vi "ProcessRun.vi"(5 "EndTime":timestamp, 7 "StartTime":timestamp, 8 "error in":errorcluster, 11 "ProcessRun":refnum<class "ProcessRun.lvclass">) -> (0 "error out":errorcluster, 3 "Passed":bool)   [LabVIEW 2020]
uses:
  ProligentResultProcessor/ProcessRun/ProcessRun.lvclass
  ProligentResultProcessor/ProcessRun/SetProcessRunId.vi
  ProligentResultProcessor/ProcessRun/SetProcessFullName.vi
  ProligentResultProcessor/ProcessRun/SetProcessVersion.vi
  ProligentResultProcessor/ProcessRun/SetProductUnitIdentifier.vi
  ProligentResultProcessor/ProcessRun/SetProductFullName.vi
  ProligentResultProcessor/ProcessRun/SetProcessRunStatus.vi
  ProligentResultProcessor/ProcessRun/SetProcessRunStartTime.vi
  ProligentResultProcessor/ProcessRun/SetProcessRunEndTime.vi
  ProligentResultProcessor/ProcessRun/SetProcessMode.vi
  ProligentResultProcessor/ProcessRun/GetProcessRunId.vi
  ProligentResultProcessor/ProcessRun/GetProcessFullName.vi
  ProligentResultProcessor/ProcessRun/GetProcessVersion.vi
  ProligentResultProcessor/ProcessRun/GetProductUnitIdentifier.vi
  ProligentResultProcessor/ProcessRun/GetProductFullName.vi
  ProligentResultProcessor/ProcessRun/GetProcessRunStatus.vi
  ProligentResultProcessor/ProcessRun/GetProcessRunStartTime.vi
  ProligentResultProcessor/ProcessRun/GetProcessRunEndTime.vi
  ProligentResultProcessor/ProcessRun/GetProcessMode.vi
  ProligentResultProcessor/ProcessRun/GetOperationRuns.vi
  ProligentResultProcessor/ProcessRun/GetOperationCycles.vi
  ProligentResultProcessor/ProcessRun/GetFailureReferences.vi
  ProligentResultProcessor/ProcessRun/GetCustomData.vi
  ProligentResultProcessor/OperationRun/OperationRun.lvclass
  ProligentResultProcessor/OperationCycle/OperationCycle.lvclass
  ProligentResultProcessor/Failure/FailureReference/FailureReference.lvclass
  ProligentResultProcessor/Model/CustomData/CustomData.lvclass
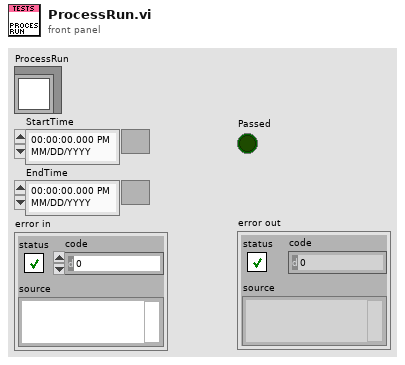
[diagram p1: front panel]
types:
  T1 = enum16{"PASS", "FAIL", "NOT_COMPLETED", "ABORTED"}
  T2 = typedef "ProligentResultProcessor.lvlib/ExecutionStatus.lvclass/Value.ctl" = enum16{"PASS", "FAIL", "NOT_COMPLETED", "ABORTED"}
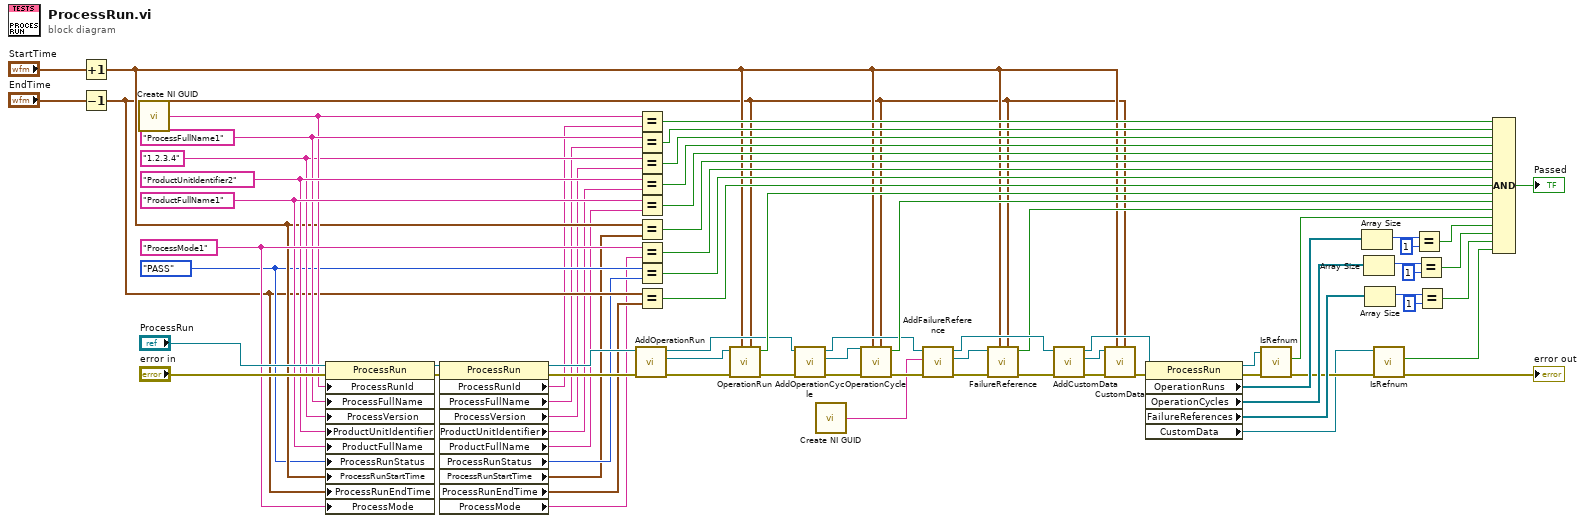
[diagram p0: block diagram]
diagram:
  w46 = "1.2.3.4"
  w27 = T1."PASS" ("ProcessRunStatus")
  w73 = "ProcessMode1"
  w72 = "ProductFullName1"
  w71 = "ProductUnitIdentifier2"
  w70 = "ProcessFullName1"
  n1 = Increment(x="StartTime") -> (x+1=w29:timestamp)
  n2 = Decrement(x="EndTime") -> (x-1=w26:timestamp)
  n3 = call <vilib>:"Create NI GUID.vi"() -> ("NI GUID"=w48:string)
  n4 = property class="ProcessRun"(reference="ProcessRun", error in="error in", "ProcessRunId"=w48, "ProcessFullName"=w70, "ProcessVersion"=w46, "ProductUnitIdentifier"=w71, "ProductFullName"=w72, "ProcessRunStatus"=w27, "ProcessRunStartTime"=w29, "ProcessRunEndTime"=w26, "ProcessMode"=w73) -> (reference out=w25:refnum<class "ProcessRun.lvclass">, error out=w24:errorcluster)
  n5 = property class="ProcessRun"(reference=w25, error in=w24) -> (reference out=w22:refnum<class "ProcessRun.lvclass">, error out=w23:errorcluster, "ProcessRunId"=w21:string, "ProcessFullName"=w20:string, "ProcessVersion"=w19:string, "ProductUnitIdentifier"=w18:string, "ProductFullName"=w17:string, "ProcessRunStatus"=w16:T2, "ProcessRunStartTime"=w15:timestamp, "ProcessRunEndTime"=w14:timestamp, "ProcessMode"=w13:string)
  n6 = call "AddOperationRun.vi"("error in"=w23, "ProcessRun in"=w22) -> ("error out"=w55:errorcluster, "OperationRun"=w56:refnum<class "OperationRun.lvclass">, "ProcessRun out"=w40:refnum<class "ProcessRun.lvclass">)  [unwired: 7 in]
  n7 = Equal?(x=w48, y=w21) -> (x = y?=w49:bool)
  n8 = Equal?(x=w70, y=w20) -> (x = y?=w65:bool)
  n9 = Equal?(x=w46, y=w19) -> (x = y?=w47:bool)
  n10 = Equal?(x=w71, y=w18) -> (x = y?=w64:bool)
  n11 = Equal?(x=w72, y=w17) -> (x = y?=w63:bool)
  n12 = Equal?(x=w29, y=w15) -> (x = y?=w62:bool)
  n13 = Equal?(x=w73, y=w13) -> (x = y?=w61:bool)
  n14 = Equal?(x=w27, y=w16) -> (x = y?=w60:bool)
  n15 = Equal?(x=w26, y=w14) -> (x = y?=w59:bool)
  n16 = call "OperationRun.vi"("EndTime"=w26, "StartTime"=w29, "error in"=w55, "OperationRun"=w56) -> ("error out"=w41:errorcluster, "Passed"=w54:bool)  [unwired: 6 in]
  n17 = call "AddOperationCycle.vi"("error in"=w41, "ProcessRun in"=w40) -> ("error out"=w39:errorcluster, "OperationRun"=w38:refnum<class "OperationCycle.lvclass">, "ProcessRun out"=w35:refnum<class "ProcessRun.lvclass">)  [unwired: 7 in]
  n18 = call <vilib>:"Create NI GUID.vi"() -> ("NI GUID"=w28:string)
  n19 = call "OperationCycle.vi"("EndTime"=w26, "StartTime"=w29, "error in"=w39, "OperationRun"=w38) -> ("error out"=w36:errorcluster, "Passed"=w37:bool)  [unwired: 6 in]
  n20 = call "AddFailureReference.vi"("error in"=w36, "Id"=w28, "ProcessRun in"=w35) -> ("error out"=w33:errorcluster, "OperationRun"=w31:refnum<class "FailureReference.lvclass">, "ProcessRun out"=w34:refnum<class "ProcessRun.lvclass">)  [unwired: 6 in]
  n21 = call "FailureReference.vi"("EndTime"=w26, "StartTime"=w29, "error in"=w33, "Defect"=w31) -> ("error out"=w32:errorcluster, "Passed"=w30:bool)  [unwired: 6 in]
  n22 = call "AddCustomData.vi"("error in"=w32, "Defect in"=w34) -> ("error out"=w45:errorcluster, "CustomData"=w44:refnum<class "CustomData.lvclass">, "Defect out"=w43:refnum<class "ProcessRun.lvclass">)  [unwired: 7 in]
  n23 = call "CustomData.vi"("EndTime"=w26, "StartTime"=w29, "error in"=w45, "CustomData"=w44) -> ("error out"=w42:errorcluster)  [unwired: 6 in, 1 out]
  n24 = property class="ProcessRun"(reference=w43, error in=w42) -> (reference out=w51:refnum<class "ProcessRun.lvclass">, error out=w66:errorcluster, "OperationRuns"=w67:refnum<class "OperationRun.lvclass">[], "OperationCycles"=w8:refnum<class "OperationCycle.lvclass">[], "FailureReferences"=w7:refnum<class "FailureReference.lvclass">[], "CustomData"=w2:refnum<class "CustomData.lvclass">)
  n25 = call "IsRefnum.vi"("error in"=w66, "ProcessRun in"=w51) -> ("error out"=w4:errorcluster, "IsRefnum"=w50:bool)  [unwired: 7 in, 1 out]
  n26 = Array Size(array=w67) -> (size(s)=w69:i32)
  n27 = Array Size(array=w8) -> (size(s)=w11:i32)
  n28 = Array Size(array=w7) -> (size(s)=w10:i32)
  n29 = call "IsRefnum.vi"("error in"=w4, "CustomDataType in"=w2) -> ("error out"=→"error out":errorcluster, "IsRefnum"=w1:bool)  [unwired: 7 in, 1 out]
  n30 = Equal?(x=w69, y=1) -> (x = y?=w58:bool)
  n31 = Equal?(x=w11, y=1) -> (x = y?=w6:bool)
  n32 = Equal?(x=w10, y=1) -> (x = y?=w5:bool)
  n33 = Compound Arithmetic op=AND(w49, w65, w47, w64, w63, w62, w61, w60, w59, w54, w37, w30, w50, w58, w6, w5, w1) -> (→"Passed":bool)
